vi "Get Category.vi"(8 "error in (no error)":errorcluster, 11 "DAQmx Watchdog editor node in":refnum<class "DAQmx Watchdog editor node.lvclass">) -> (0 "error out":errorcluster, 2 "Category":string, 3 "DAQmx Watchdog editor node out":refnum<class "DAQmx Watchdog editor node.lvclass">)   [LabVIEW 2014, in "DAQmx Watchdog editor node.lvclass"]
uses:
  DAQmx Watchdog editor node.lvclass
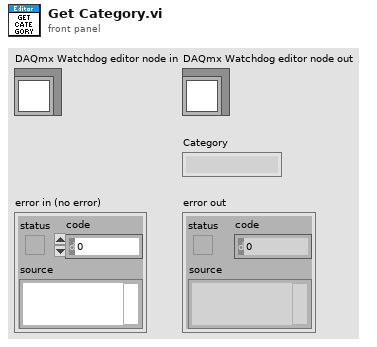
[diagram p1: front panel]
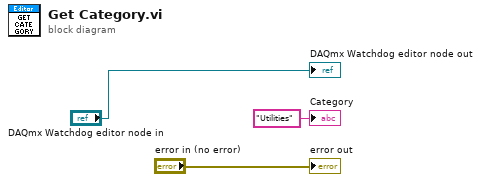
[diagram p0: block diagram]
diagram:
  "error out" <- "error in (no error)"
  "DAQmx Watchdog editor node out" <- "DAQmx Watchdog editor node in"
  "Category" <- "Utilities" ("Category")
